vi "Connection_example.vi"() -> ()   [LabVIEW 2022 SP3]
uses:
  <vilib>/addons/_JKI.lib/_JKI_lib_TCP_Server.llb/TCP Server Public Connections Info Cluster.ctl
  <vilib>/addons/_jki/python_bridge/Server/Server.lvclass
  <vilib>/addons/_JKI.lib/_JKI_lib_TCP_Server.llb/JKI TCP Server.lvclass
panel:
  out "error out":errorcluster
  out "Number of Connections":u32
  out "Client Connected":bool
  out "Connections Info":T1[](array[typedef])
  in  "stop":bool
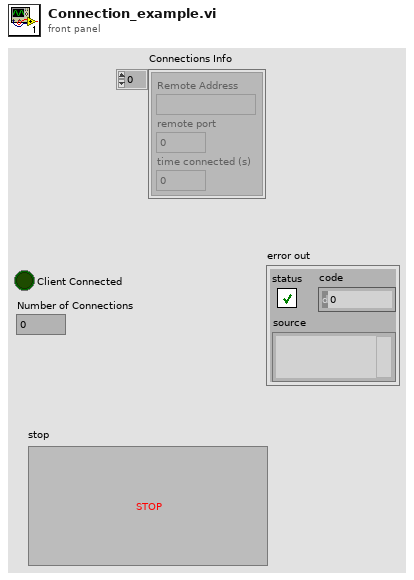
[diagram p1: front panel]
types:
  T1 = typedef "JKI TCP Server.lvclass/TCP Server Public Connections Info Cluster.ctl" = cluster{"Remote Address":string, "remote port":u16, "time connected (s)":dbl}
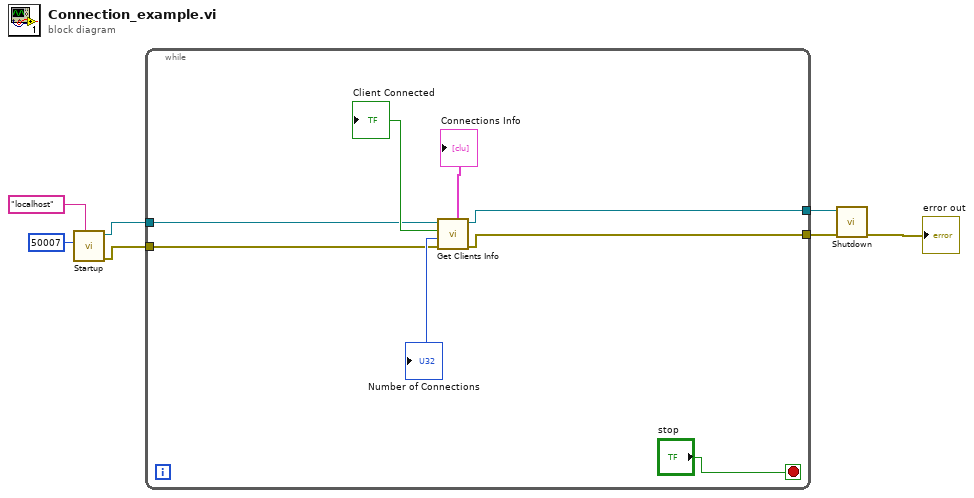
[diagram p0: block diagram]
diagram:
  n1 = call <vilib>:"Startup.vi"("IP Address (localhost)"="localhost", "TCP port (50007)"=u16 50007) -> ("error out"=w5:errorcluster, "JKI_Python_Server out"=w4:refnum<class "Server.lvclass">)  [unwired: 8 in]
  n2 = while {
    tunnel: w5 -> [w11]
    tunnel: w4 -> [w10]
    tunnel: [w9] -> w2
    tunnel: [w8] -> w1
    stop <- "stop" stop-if-true
    n3 = call <vilib>:"Get Clients Info.vi"("error in (no error)"=w11, "JKI_Python_Server in"=w10) -> ("error out"=w9:errorcluster, "Number of Connections"=→"Number of Connections":u32, "Client Connected"=→"Client Connected":bool, "JKI_Python_Server out"=w8:refnum<class "Server.lvclass">, "Connections Info"=→"Connections Info":T1[])  [unwired: 5 in]
  }
  n4 = call <vilib>:"Shutdown.vi"("error in (no error)"=w2, "JKI_Python_Server in"=w1) -> ("error out"=→"error out":errorcluster)  [unwired: 9 in]
